vi "Teardown Init.vi"(8 "Error in":errorcluster, 11 "TEMPLATE Actor in":refnum<class "TEMPLATE Actor.lvclass">) -> ()   [LabVIEW 2025, in "TEMPLATE Actor.lvlib" / "TEMPLATE Actor.lvclass"]
uses:
  TEMPLATE Actor.lvclass
  TEMPLATE Actor.lvclass/TEMPLATE Actor.ctl
  <vilib>/Nathan Davis/jettl/jettl/jettl/Actor/Actor/Actor.lvclass
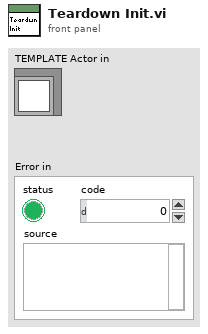
[diagram p1: front panel]
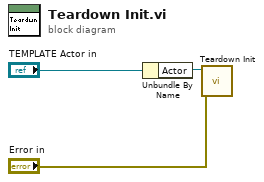
[diagram p0: block diagram]
diagram:
  n1 = Unbundle By Name("TEMPLATE Actor in") -> ("Actor"=w1:refnum<class "Actor.lvclass">)
  n2 = call-dynamic "Teardown Init.vi"("Error in"="Error in", "Actor in"=w1) -> ()  [unwired: 10 in]
